vi "HMI_Example.vi"() -> ()   [LabVIEW 2017, in "Examples.lvlib"]
uses:
  Examples.lvlib
panel:
  in  "Boolean":bool
  in  "Fan":bool
  in  "Mixer":bool
  out "Valve":bool
  in  "Boiler":bool
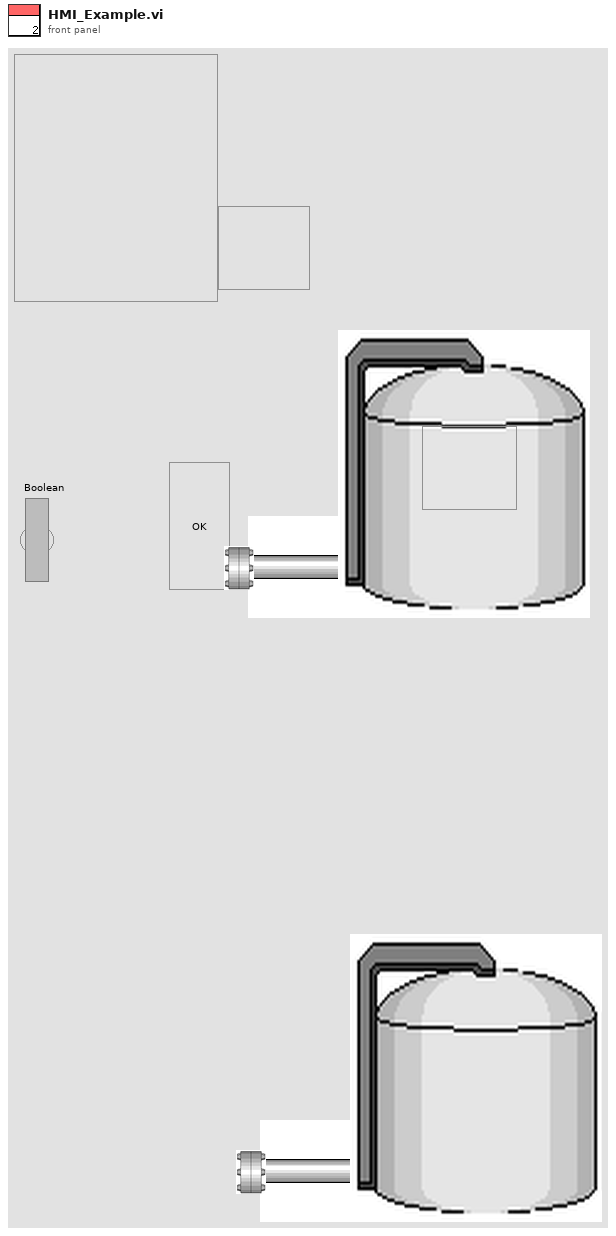
[diagram p1: front panel]
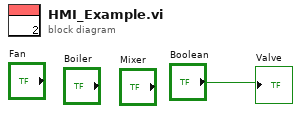
[diagram p0: block diagram]
diagram:
  "Valve" <- "Boolean"
